vi "Index Array.vi"() -> ()   [LabVIEW 2017]
panel:
  out "Element":string
  in  "Array":string[](array[string])
  out "Element":dbl
  # "Index Array Examples"
  # "See the Block Diagram!"
  # "The 0th Element is the First Value"
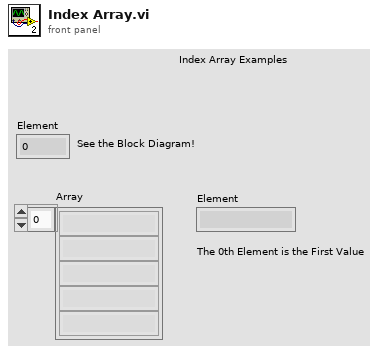
[diagram p1: front panel]
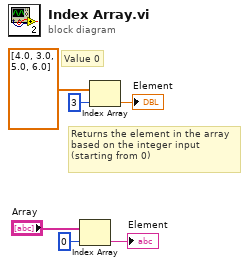
[diagram p0: block diagram]
diagram:
  # "Value 0"
  # "Returns the element in the array\nbased on the integer input\n(starting from 0)"
  n1 = Index Array(array="Array", index=0) -> (element=→"Element":string)
  n2 = Index Array(array=dbl[] [4.0, 3.0, 5.0, 6.0], index=3) -> (element=→"Element":dbl)
